vi "Test Cluster.vi"() -> ()   [LabVIEW 2015]
panel:
  in  "?":T1
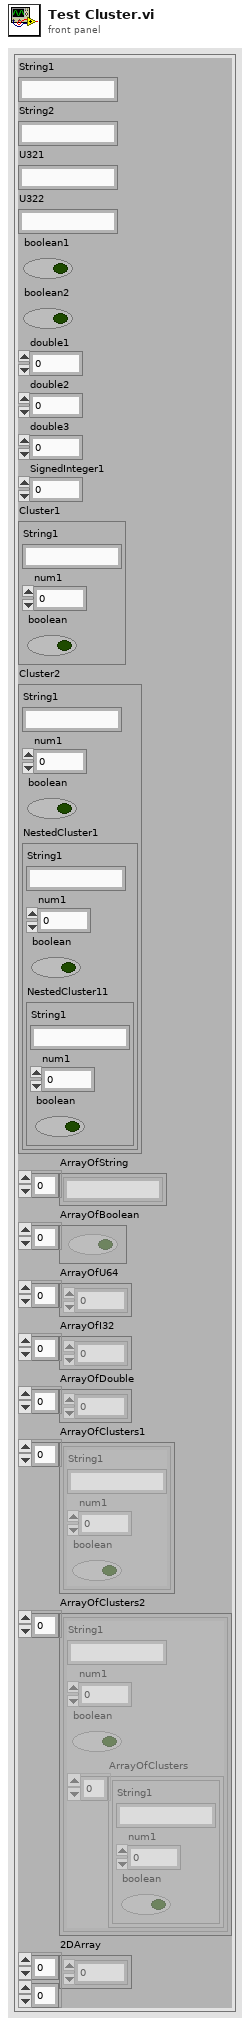
[diagram p1: front panel]
types:
  T1 = cluster{"String1":string, "String2":string, "U321":string, "U322":string, "boolean1":bool, "boolean2":bool, "double1":dbl, "double2":dbl, "double3":i64, "SignedInteger1":i64, "Cluster1":cluster{"String1":string, "num1":dbl, "boolean":bool}, "Cluster2":cluster{"String1":string, "num1":dbl, "boolean":bool, "NestedCluster1":cluster{"String1":string, "num1":dbl, "boolean":bool, "NestedCluster11":cluster{"String1":string, "num1":dbl, "boolean":bool}}}, "ArrayOfString":string[], "ArrayOfBoolean":bool[], "ArrayOfU64":i32[], "ArrayOfI32":i32[], "ArrayOfDouble":i32[], "ArrayOfClusters1":cluster{"String1":string, "num1":dbl, "boolean":bool}[], "ArrayOfClusters2":cluster{"String1":string, "num1":dbl, "boolean":bool, "ArrayOfClusters":cluster{"String1":string, "num1":dbl, "boolean":bool}[]}[], "2DArray":i32[][]}
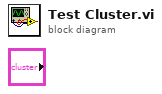
[diagram p0: block diagram]
diagram:
